vi "FPGA Main.vi"() -> ()   [LabVIEW 2013]
uses:
  dynamic profibus/profibus master action.ctl
  dynamic profibus/profibus master transmit state.ctl
  dynamic profibus/profibus master transmit header.ctl
  <vilib>/rvi/Emulation/niFpgaSctlEmulationGetInTimedLoop.vi
  <vilib>/rvi/Emulation/niFpgaEmulationReportErrorSimple.vi
  <vilib>/rvi/Emulation/niFpgaGetClockAttributes.vi
  <vilib>/rvi/DataTransferAndStorage/Container/Common/niFpgaContainerGetUniqueNameForEmu.vi
  <vilib>/rvi/DataTransferAndStorage/Container/Common/niFpgaContainerSetEmuInfo.vi
  <vilib>/rvi/eio/common/nirviEmuReportErrorAndStop.vi
  <vilib>/rvi/eio/common/nirviEmuTemplatePropertySet_errors.vi
  <vilib>/rvi/Emulation/niFpgaCriticalErrorInLSC.vi
  <vilib>/rvi/eio/common/nirviEmuTemplateMethod_errors.vi
  <vilib>/rvi/DataTransferAndStorage/Container/Common/niFpgaContainerExecOnDevCompGetState.vi
  <vilib>/rvi/FIFO/Fifo_Resource/nirvififoEmulationReadFpgaImpl.vi
  <vilib>/rvi/interface/RandomDataEmulation/nirviRandomDataFPGAFIFO.vi
  <vilib>/rvi/interface/RandomDataEmulation/niFpgaRandomDataHandleErrors.vi
  <vilib>/rvi/Memory/Memory_Emulation/nirvimemoryFastEmulationFpgaImpl.vi
  <instcachedir>/0/nirvimemoryFastEmulationFpgaImpl_5FBAB50466BC4C939F684F8805638BFC.lvgen/nirvimemoryFastEmulationFpgaImpl_5FBAB50466BC4C939F684F8805638BFC_002.vi
  <vilib>/rvi/Memory/Memory_Emulation/niFpgaMemoryEmulationCacheClearOnFirstRun.vi
  <vilib>/rvi/Memory/Memory_Emulation/nirvimemoryEmulationManagerCache_MakeExclusive.vi
  <vilib>/rvi/Memory/Memory_Emulation/niFpgaMemoryEmulationValidateCache.vi
  <vilib>/rvi/Memory/Memory_Emulation/nirvimemoryEmulationManagerCache_ReleaseExclusive.vi
  <vilib>/rvi/Memory/Memory_Emulation/nirvimemoryEmulationManagerCache_InsertValue.vi
  <vilib>/Utility/error.llb/Clear Errors.vi
  <vilib>/rvi/Memory/Memory_Emulation/nirvimemoryEmulationManagerCache_SetValue.vi
  <vilib>/rvi/Emulation/niFpgaSctlEmulationResourceMgr.vi
  <vilib>/rvi/Emulation/niFpgaProcessEmulError.vi
  <vilib>/rvi/Memory/Memory_Emulation/nirvimemoryEmulationManagerCache_GetValue.vi
  <vilib>/rvi/FIFO/Fifo_Resource/nirvififoEmulationWriteFpgaImpl.vi
  <vilib>/rvi/LocalResourceManager/LocalResourceManager.xnode
  <vilib>/eio/EIOPropertyNode/EIOPropertyNode.xnode
  <vilib>/eio/EIOMethodNode/EIOMethodNode.xnode
  <vilib>/rvi/DataTransferAndStorage/Container/XNode/niFpgaContainer.xnode
  <vilib>/rvi/FIFO/Fifo_Resource/niFpgaFifoEmulationRefIn.vi
  <vilib>/rvi/Memory/Memory_Emulation/niFpgaMemoryEmulationRefIn.vi
  <vilib>/rvi/eio/common/nirviEmuTemplatePropertyGet_errors.vi
  <vilib>/rvi/eio/common/nirviEmuTemplatePropertyGet_noerrors.vi
  <vilib>/rvi/eio/common/nirviEmuTemplatePropertySet_noerrors.vi
panel:
  out "wait to start":bool
  in  "start":bool
  in  "stop":bool
  out "ready":bool
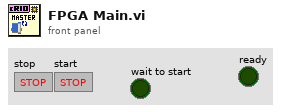
[diagram p1: front panel]
types:
  T1 = typedef "profibus master transmit state.ctl" = enum16{"Check IO", "DP Transfer", "Send Input Count", "Send Inputs", "Check Diagnostic", "Diagnostic Transfer", "Send Diagnostic Count", "Send Diagnostics", "Next Slave", "Finalize"}
  T2 = typedef "profibus master transmit header.ctl" = enum8{"Input", "Diagnostic"}
  T3 = typedef "profibus master action.ctl" = enum8{"set output", "transfer complete", "configure reads", "configure diagnostics"}
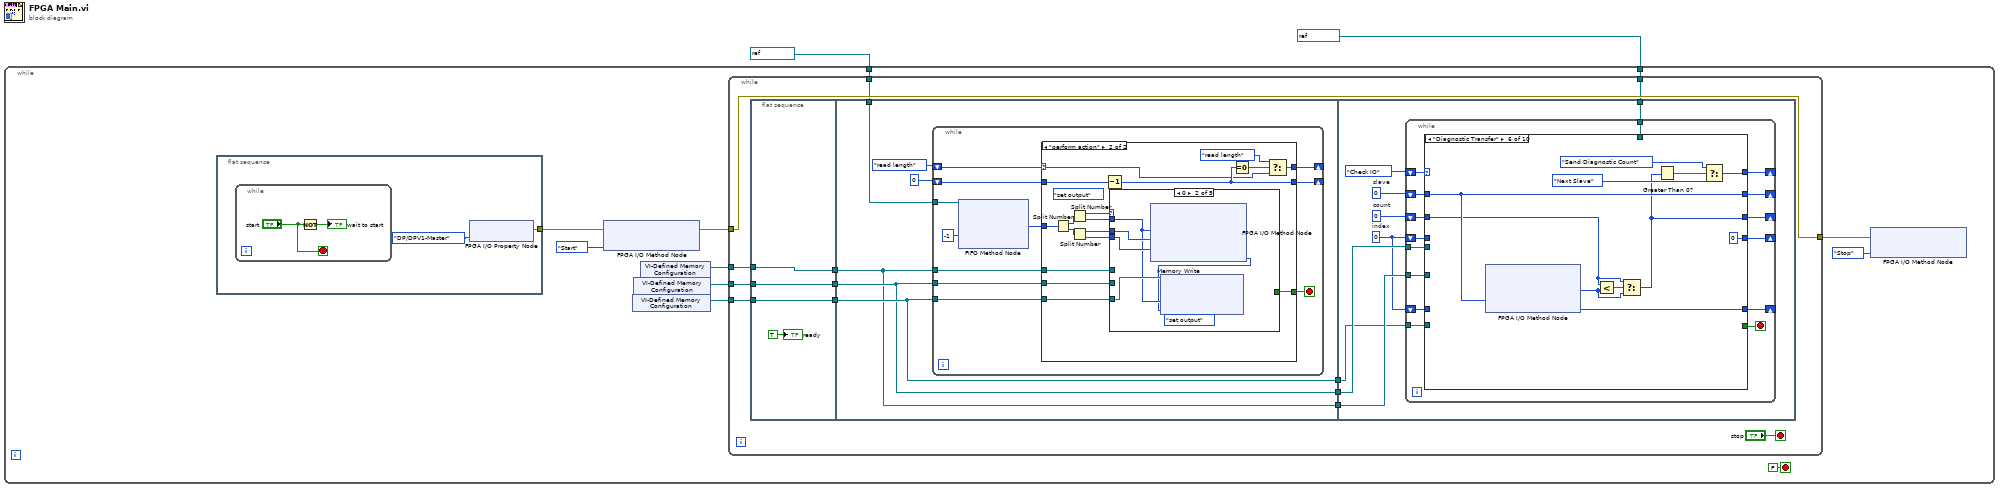
[diagram p0: block diagram]
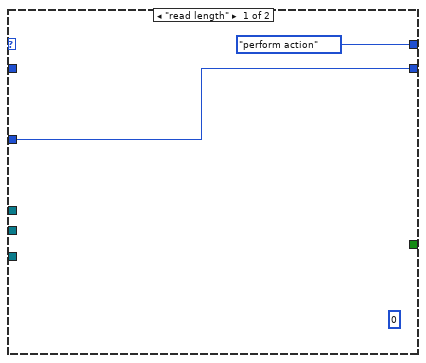
[diagram p2: hidden frame]
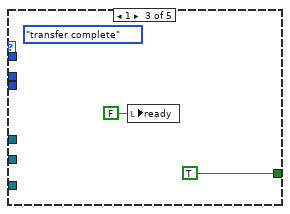
[diagram p4: hidden frame]
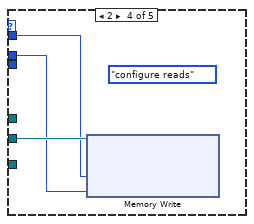
[diagram p5: hidden frame]
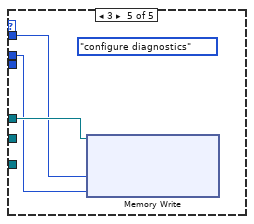
[diagram p6: hidden frame]
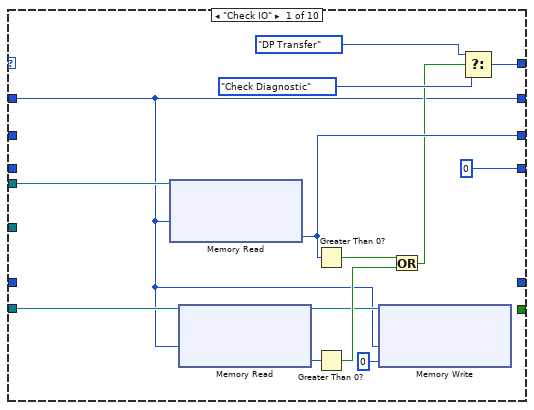
[diagram p7: hidden frame]
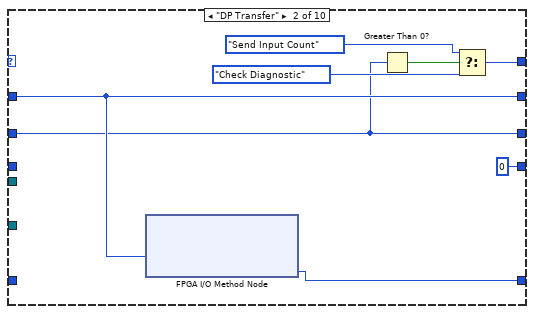
[diagram p8: hidden frame]
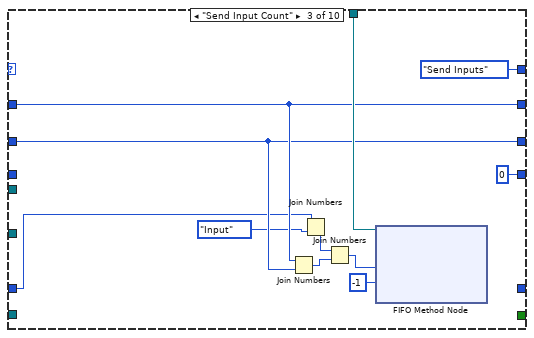
[diagram p9: hidden frame]
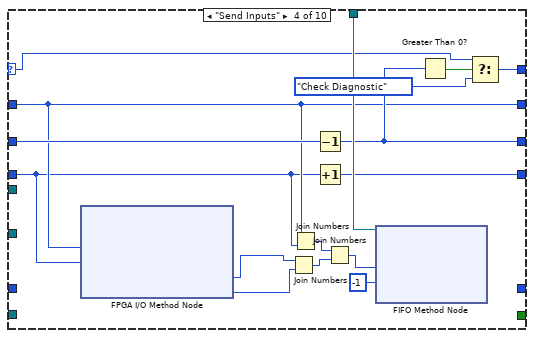
[diagram p10: hidden frame]
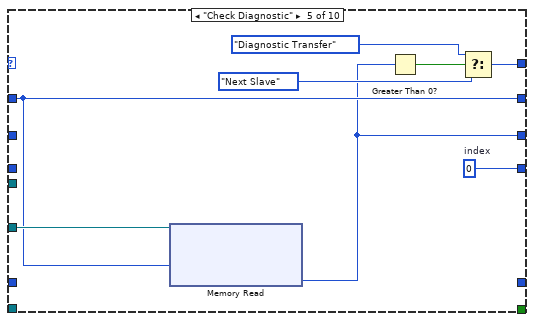
[diagram p11: hidden frame]
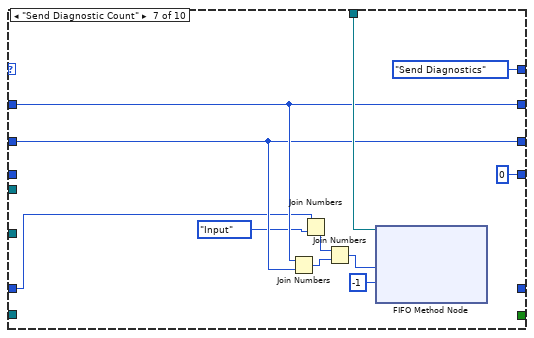
[diagram p12: hidden frame]
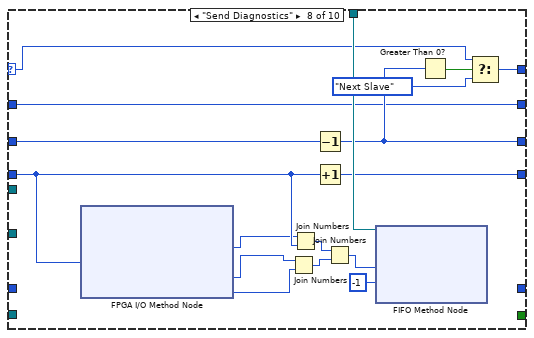
[diagram p13: hidden frame]
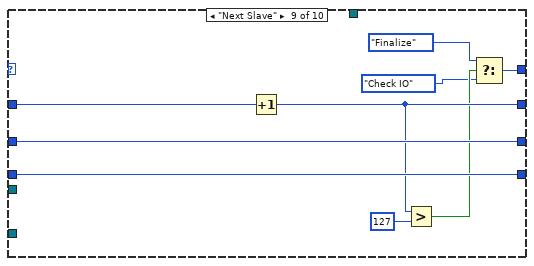
[diagram p14: hidden frame]
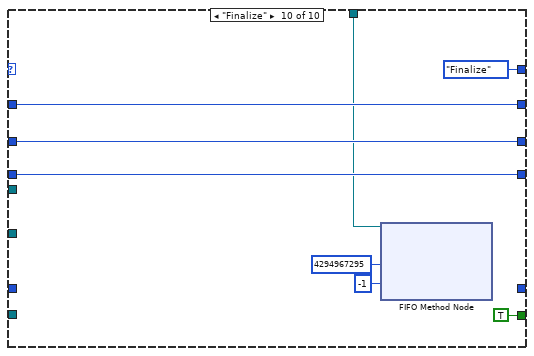
[diagram p15: hidden frame]
diagram:
  n1 = while {
    tunnel: refnum<k21> "ToHost" ("FIFO In") -> [w4]
    tunnel: refnum<k21> "ToFPGA" ("FIFO In") -> [w3]
    stop <- FALSE ("stop 2") stop-if-true
    n2 = flat-sequence {
      tunnel: [w14] -> w12
      frame #0 {
        n3 = while {
          stop <- "start" stop-if-true
          n4 = Not(x="start") -> (.not. x?=→"wait to start":bool)
        }
        n5 = xnode "FPGA I/O Property Node"("Init cRIO PB"=enum8{"DP/DPV1-Master", "DP-AutoSlave"}."DP/DPV1-Master" ("Start-up cRIO PB")) -> ("error out"=w14:errorcluster)  [unwired: 2 in, 1 out]
      }
    }
    n6 = xnode "FPGA I/O Method Node"("error in"=w12, "Mode"=enum16{"Start", "Stop"}."Start") -> ("error out"=w9:errorcluster)  [unwired: 1 in, 1 out]
    n7 = xnode ("VI-Defined Memory Configuration")() -> ("Memory Out"=w7:refnum<k21>)
    n8 = xnode ("VI-Defined Memory Configuration")() -> ("Memory Out"=w8:refnum<k21>)
    n9 = xnode ("VI-Defined Memory Configuration")() -> ("Memory Out"=w6:refnum<k21>)
    n10 = while {
      tunnel: w9 -> [w30]
      tunnel: [w30] -> w10
      tunnel: w8 -> [w28]
      tunnel: w7 -> [w27]
      tunnel: w6 -> [w24]
      tunnel: w4 -> [w22]
      tunnel: w3 -> [w18]
      stop <- "stop" stop-if-true
      n11 = flat-sequence {
        tunnel: [w34] -> w29
        tunnel: w28 -> [w34]
        tunnel: w27 -> [w33]
        tunnel: [w33] -> w26
        tunnel: [w32] -> w25
        tunnel: w24 -> [w32]
        tunnel: w29 -> [w37]
        tunnel: w26 -> [w38]
        tunnel: w25 -> [w36]
        tunnel: [w38] -> w21
        tunnel: [w37] -> w20
        tunnel: [w36] -> w19
        tunnel: w18 -> [w35]
        tunnel: w20 -> [w88]
        tunnel: w19 -> [w87]
        tunnel: w22 -> [w86]
        tunnel: w21 -> [w85]
        frame #0 {
          "ready" <- TRUE ("ready")
        }
        frame #1 {
          n12 = while {
            tunnel: w35 -> [w50]
            shift-right: [w48] -> _
            shift-left: enum16{"read length", "perform action"}."read length" -> [w49]
            shift-right: [w45] -> _
            shift-left: u32 0 -> [w47]
            tunnel: w37 -> [w43]
            tunnel: w38 -> [w42]
            tunnel: w36 -> [w41]
            stop <- w44 stop-if-true
            n13 = xnode ("FIFO Method Node")("Timeout"=-1, "FIFO In"=w50) -> ("Element"=w46:u32)  [unwired: 2 out]
            n14 = case shown="\"perform action\"" w49 {
              selector: w49 -> [_ w58]
              tunnel: [enum16{"read length", "perform action"}."perform action" w61] -> w48
              tunnel: w47 -> [_ w70]
              tunnel: [w52 w62] -> w45
              tunnel: w46 -> [w52 w57]
              tunnel: [_ w64] -> w44
              tunnel: w43 -> [_ w63]
              tunnel: w42 -> [_ w56]
              tunnel: w41 -> [_ w55]
              frame "read length" {
                (unwired) u32 0
              }
              frame "perform action" {
                (unwired) profibus_master_action."set output" ("action")
                n15 = Split Number(x=w57) -> (hi(x)=w69:u16, lo(x)=w68:u16)
                n16 = Split Number(x=w69) -> (hi(x)=w54:u8, lo(x)=w67:u8)
                n17 = Split Number(x=w68) -> (hi(x)=w66:u8, lo(x)=w65:u8)
                n18 = Decrement(x=w70) -> (x-1=w62:u32)
                n19 = case shown="0" w54 {
                  tunnel: w67 -> [_ w72 _ w79 w82]
                  tunnel: w66 -> [_ w75 _ w78 w81]
                  tunnel: w65 -> [_ w74 _ _ _]
                  tunnel: [_ _ TRUE _ _] -> w64
                  tunnel: w63 -> [_ _ _ w80 _]
                  tunnel: w56 -> [_ w73 _ _ _]
                  tunnel: w55 -> [_ _ _ _ w83]
                  frame Default {
                  }
                  frame 0 {
                    (unwired) profibus_master_action."set output" ("action")
                    n20 = xnode "FPGA I/O Method Node"("Slave"=w72, "Index"=w75, "Data"=w74) -> ("Length"=w71:u8)  [unwired: 1 in, 1 out]
                    n21 = xnode ("Memory Write")("Address"=w72, "Data"=w71, "Memory In"=w73) -> ()  [unwired: 1 out]
                  }
                  frame 1 {
                    (unwired) profibus_master_action."transfer complete" ("action")
                    n22 = local write "ready"(FALSE ("ready")) -> ()
                  }
                  frame 2 {
                    (unwired) profibus_master_action."configure reads" ("action")
                    n23 = xnode ("Memory Write")("Address"=w79, "Data"=w78, "Memory In"=w80) -> ()  [unwired: 1 out]
                  }
                  frame 3 {
                    (unwired) profibus_master_action."configure diagnostics" ("action")
                    n24 = xnode ("Memory Write")("Address"=w82, "Data"=w81, "Memory In"=w83) -> ()  [unwired: 1 out]
                  }
                }
                n25 = Equal To 0?(x=w62) -> (x = 0?=w60:bool)
                n26 = Select(t=enum16{"read length", "perform action"}."read length", s=w60, f=w58) -> (s? t:f=w61:enum16{"read length", "perform action"})
              }
            }
          }
        }
        frame #2 {
          w84 = u8 0  # index
          w89 = u8 0  # count
          w91 = u8 0  # slave
          n27 = while {
            shift-right: [w98] -> _
            shift-left: w91 -> [w105]
            shift-right: [w100] -> _
            shift-left: profibus_master_transmit_state."Check IO" -> [w106]
            shift-right: [w99] -> _
            shift-left: w89 -> [w104]
            tunnel: w88 -> [w103]
            tunnel: w87 -> [w102]
            tunnel: w86 -> [w101]
            shift-right: [w97] -> _
            shift-left: w84 -> [w96]
            tunnel: w85 -> [w95]
            shift-right: [w93] -> _
            shift-left: w84 -> [w92]
            stop <- w94 stop-if-true
            n28 = case shown="\"Diagnostic Transfer\"" w106 {
              selector: w106 -> [_ _ _ w141 _ _ _ w188 _ _]
              tunnel: w105 -> [w107 w128 w133 w144 w158 w169 w179 w191 w210 w218]
              tunnel: w104 -> [_ w123 w132 w151 _ w166 w178 w198 w211 w219]
              tunnel: w103 -> [w120 _ _ _ _ _ _ _ _ _]
              tunnel: w102 -> [_ _ _ _ w159 _ _ _ _ _]
              tunnel: w101 -> [_ _ w138 w155 _ _ w184 w202 _ w215]
              tunnel: [w119 w125 profibus_master_transmit_state."Send Inputs" w147 w162 w172 profibus_master_transmit_state."Send Diagnostics" w194 w203 profibus_master_transmit_state."Finalize"] -> w100
              tunnel: [w118 w123 w132 w148 w157 w165 w178 w195 w211 w219] -> w99
              tunnel: [w107 w128 w133 w144 w158 w169 w179 w191 w208 w218] -> w98
              tunnel: [u8 0 ("index") u8 0 ("index") u8 0 ("index") w150 w156 u8 0 ("index") u8 0 ("index") w197 w209 w217] -> w97
              tunnel: w96 -> [_ _ _ w143 _ _ _ w190 w209 w217]
              tunnel: w95 -> [w114 _ _ _ _ _ _ _ _ _]
              tunnel: [_ _ _ _ _ _ _ _ _ TRUE] -> w94
              tunnel: [_ w121 _ _ _ w164 _ _ _ _] -> w93
              tunnel: w92 -> [_ _ w129 _ _ _ w175 _ _ _]
              frame "Check IO" {
                n29 = xnode ("Memory Read")("Address"=w107, "Memory In"=w120) -> ("Data"=w118:u8)  [unwired: 1 out]
                n30 = xnode ("Memory Read")("Address"=w107, "Memory In"=w114) -> ("Data"=w113:u8, "Memory Out"=w109:refnum<k21>)
                n31 = Greater Than 0?(x=w118) -> (x > 0?=w112:bool)
                n32 = Greater Than 0?(x=w113) -> (x > 0?=w110:bool)
                n33 = xnode ("Memory Write")("Address"=w107, "Data"=u8 0, "Memory In"=w109) -> ()  [unwired: 1 out]
                n34 = Or(x=w112, y=w110) -> (x .or. y?=w111:bool)
                n35 = Select(t=profibus_master_transmit_state."DP Transfer", s=w111, f=profibus_master_transmit_state."Check Diagnostic") -> (s? t:f=w119:T1)
              }
              frame "DP Transfer" {
                n36 = xnode "FPGA I/O Method Node"("Slave"=w128) -> ("Slave Status"=w121:u8)  [unwired: 2 in, 2 out]
                n37 = Greater Than 0?(x=w123) -> (x > 0?=w124:bool)
                n38 = Select(t=profibus_master_transmit_state."Send Input Count", s=w124, f=profibus_master_transmit_state."Check Diagnostic") -> (s? t:f=w125:T1)
              }
              frame "Send Input Count" {
                n39 = Join Numbers(hi=w133, lo=w132) -> ((hi.lo)=w135:u16)
                n40 = Join Numbers(hi=w129, lo=profibus_master_transmit_header."Input") -> ((hi.lo)=w131:u16)
                n41 = Join Numbers(hi=w131, lo=w135) -> ((hi.lo)=w134:u32)
                n42 = xnode ("FIFO Method Node")("Element"=w134, "Timeout"=-1, "FIFO In"=w138) -> ()  [unwired: 2 out]
              }
              frame "Send Inputs" {
                n43 = xnode "FPGA I/O Method Node"("Slave"=w144, "Index"=w143) -> ("Data"=w142:u8, "Length"=w140:u8)  [unwired: 2 in, 2 out]
                n44 = Join Numbers(hi=w142, lo=w140) -> ((hi.lo)=w153:u16)
                n45 = Join Numbers(hi=w144, lo=w143) -> ((hi.lo)=w145:u16)
                n46 = Decrement(x=w151) -> (x-1=w148:u8)
                n47 = Increment(x=w143) -> (x+1=w150:u8)
                n48 = Join Numbers(hi=w145, lo=w153) -> ((hi.lo)=w152:u32)
                n49 = xnode ("FIFO Method Node")("Element"=w152, "Timeout"=-1, "FIFO In"=w155) -> ()  [unwired: 2 out]
                n50 = Greater Than 0?(x=w148) -> (x > 0?=w149:bool)
                n51 = Select(t=w141, s=w149, f=profibus_master_transmit_state."Check Diagnostic") -> (s? t:f=w147:T1)
              }
              frame "Check Diagnostic" {
                w156 = u8 0  # index
                n52 = xnode ("Memory Read")("Address"=w158, "Memory In"=w159) -> ("Data"=w157:u8)  [unwired: 1 out]
                n53 = Greater Than 0?(x=w157) -> (x > 0?=w163:bool)
                n54 = Select(t=profibus_master_transmit_state."Diagnostic Transfer", s=w163, f=profibus_master_transmit_state."Next Slave") -> (s? t:f=w162:T1)
              }
              frame "Diagnostic Transfer" {
                n55 = xnode "FPGA I/O Method Node"("Slave"=w169) -> ("Read Count"=w167:u8, "Slave Status"=w164:u8)  [unwired: 2 in, 2 out]
                n56 = Less?(x=w166, y=w167) -> (x < y?=w168:bool)
                n57 = Select(t=w166, s=w168, f=w167) -> (s? t:f=w165:u8)
                n58 = Greater Than 0?(x=w165) -> (x > 0?=w171:bool)
                n59 = Select(t=profibus_master_transmit_state."Send Diagnostic Count", s=w171, f=profibus_master_transmit_state."Next Slave") -> (s? t:f=w172:T1)
              }
              frame "Send Diagnostic Count" {
                n60 = Join Numbers(hi=w179, lo=w178) -> ((hi.lo)=w181:u16)
                n61 = Join Numbers(hi=w175, lo=profibus_master_transmit_header."Input") -> ((hi.lo)=w177:u16)
                n62 = Join Numbers(hi=w177, lo=w181) -> ((hi.lo)=w180:u32)
                n63 = xnode ("FIFO Method Node")("Element"=w180, "Timeout"=-1, "FIFO In"=w184) -> ()  [unwired: 2 out]
              }
              frame "Send Diagnostics" {
                n64 = xnode "FPGA I/O Method Node"("Index"=w190) -> ("Slave"=w187:i8, "Data"=w189:u8, "Length"=w186:u8)  [unwired: 2 in, 2 out]
                n65 = Join Numbers(hi=w189, lo=w186) -> ((hi.lo)=w200:u16)
                n66 = Join Numbers(hi=w187, lo=w190) -> ((hi.lo)=w192:u16)
                n67 = Decrement(x=w198) -> (x-1=w195:u8)
                n68 = Increment(x=w190) -> (x+1=w197:u8)
                n69 = Join Numbers(hi=w192, lo=w200) -> ((hi.lo)=w199:u32)
                n70 = xnode ("FIFO Method Node")("Element"=w199, "Timeout"=-1, "FIFO In"=w202) -> ()  [unwired: 2 out]
                n71 = Greater Than 0?(x=w195) -> (x > 0?=w196:bool)
                n72 = Select(t=w188, s=w196, f=profibus_master_transmit_state."Next Slave") -> (s? t:f=w194:T1)
              }
              frame "Next Slave" {
                n73 = Increment(x=w210) -> (x+1=w208:u8)
                n74 = Greater?(x=w208, y=u8 127) -> (0:w206:bool)
                n75 = Select(t=profibus_master_transmit_state."Finalize", s=w206, f=profibus_master_transmit_state."Check IO") -> (s? t:f=w203:T1)
              }
              frame "Finalize" {
                n76 = xnode ("FIFO Method Node")("Element"=u32 4294967295, "Timeout"=-1, "FIFO In"=w215) -> ()  [unwired: 2 out]
              }
            }
          }
        }
      }
    }
    n77 = xnode "FPGA I/O Method Node"("error in"=w10, "Mode"=enum16{"Start", "Stop"}."Stop") -> ()  [unwired: 1 in, 2 out]
  }
